vi "Gen - SubPanel Page.vi"(6 "State":T1(ring), 7 "Module Name":string, 8 "Error In":errorcluster, 9 "Module List":string[](array[string]), 10 "Path to Modules Folder":path, 11 "Main SubPanel Ref":refnum<vi>) -> (0 "Error Out":errorcluster)   [LabVIEW 2020]
doc: "Use this VI to calling page and display into subpanel\n\nWriter :\nReader : Main UI"
uses:
  Control/aFGV States - Subpanel.ctl
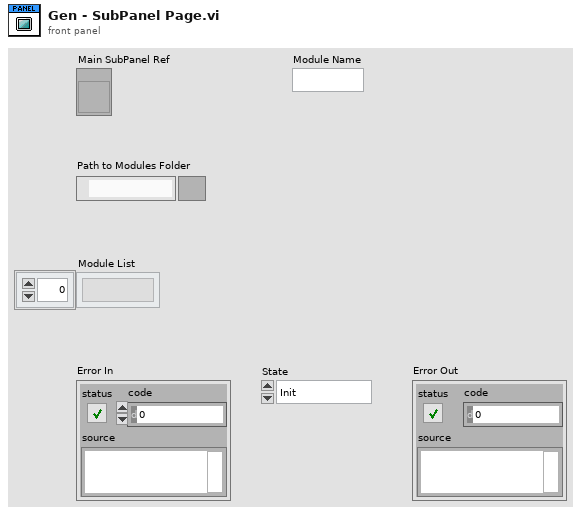
[diagram p1: front panel]
types:
  T1 = enum16{"Init", "Init Module", "Run Module", "Kill Module", "Change Page", "Exit"}
  T2 = typedef "aFGV States - Subpanel.ctl" = enum16{"Init", "Get VI Name", "Update", "Exit"}
  T3 = enum32{"Bad", "Idle", "Run top level", "Running"}
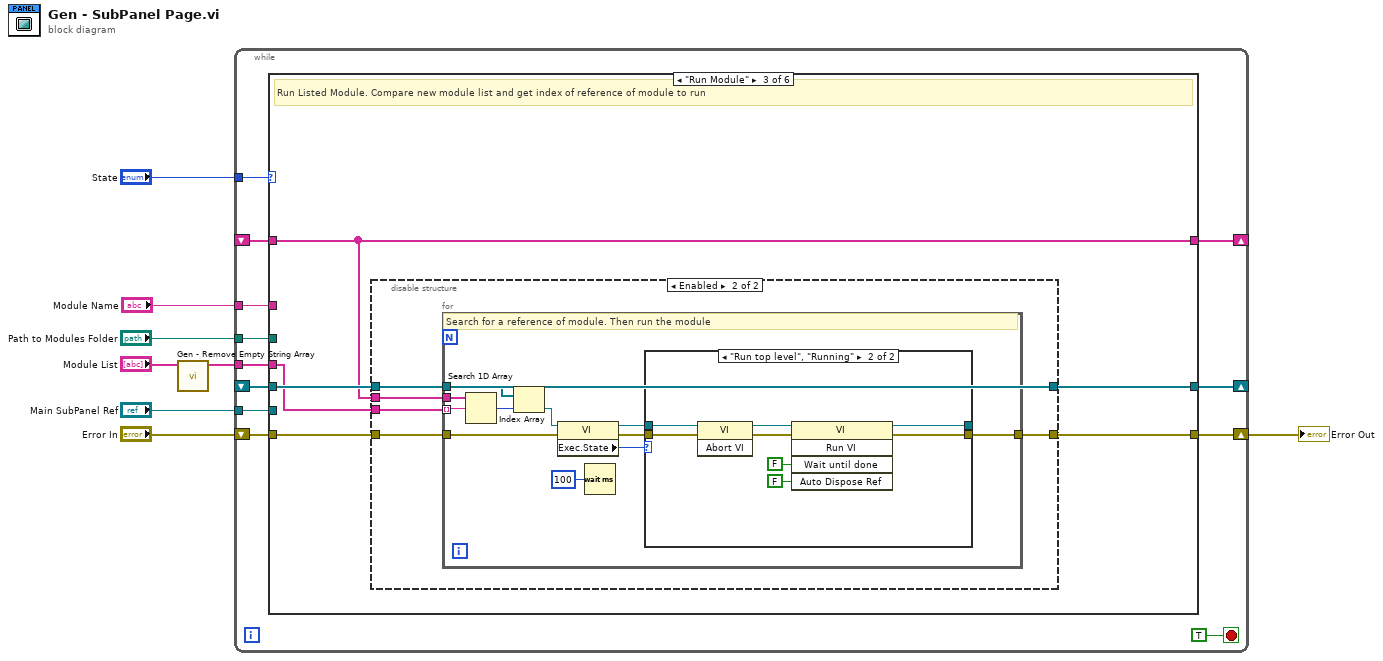
[diagram p0: block diagram]
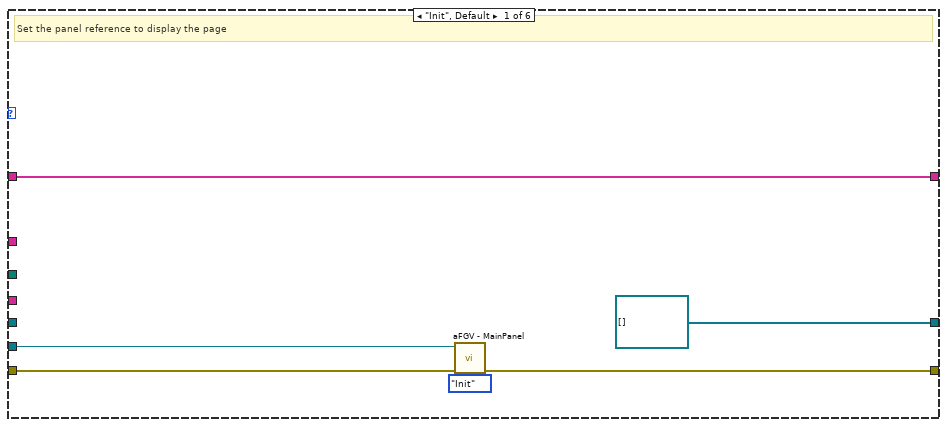
[diagram p2: hidden frame]
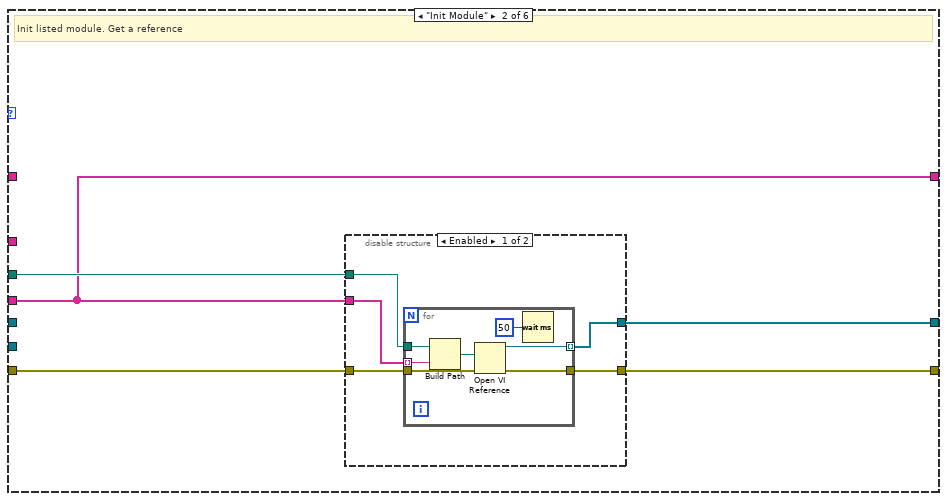
[diagram p3: hidden frame]
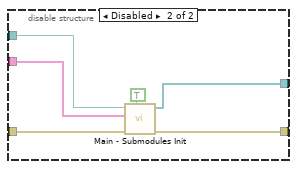
[diagram p4: hidden frame]
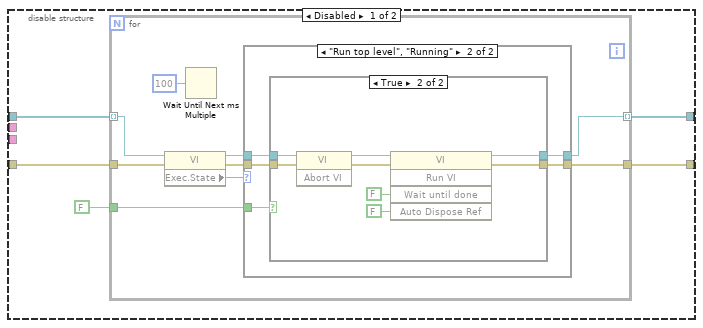
[diagram p5: hidden frame]
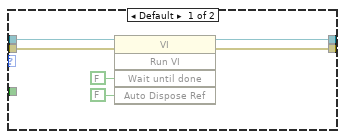
[diagram p6: hidden frame]
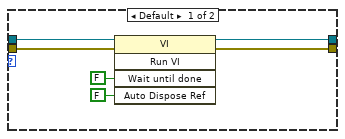
[diagram p8: hidden frame]
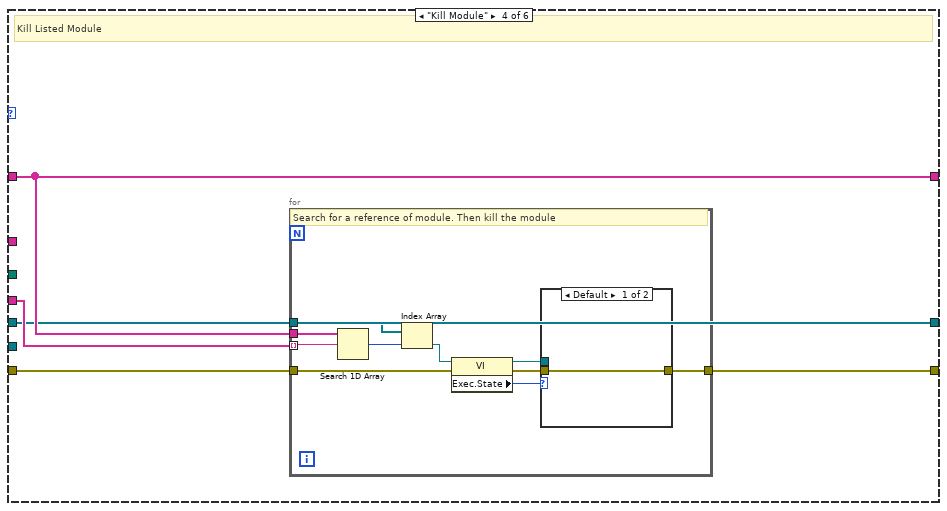
[diagram p9: hidden frame]
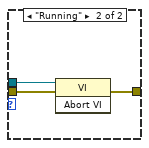
[diagram p10: hidden frame]
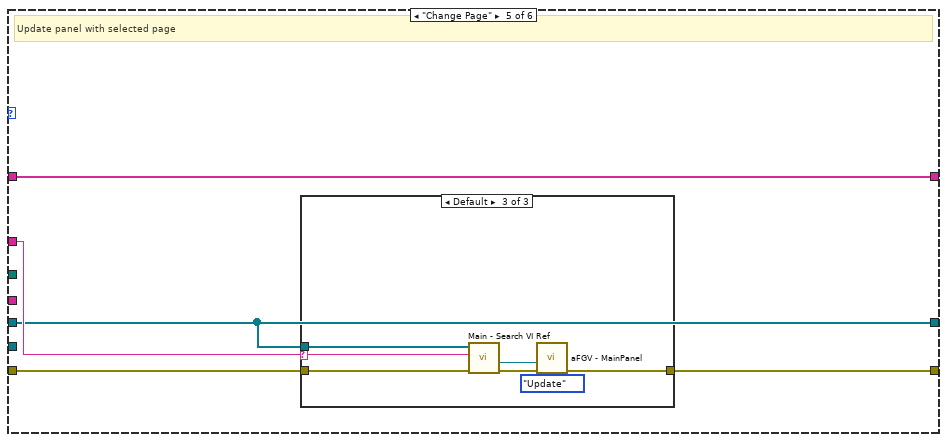
[diagram p11: hidden frame]
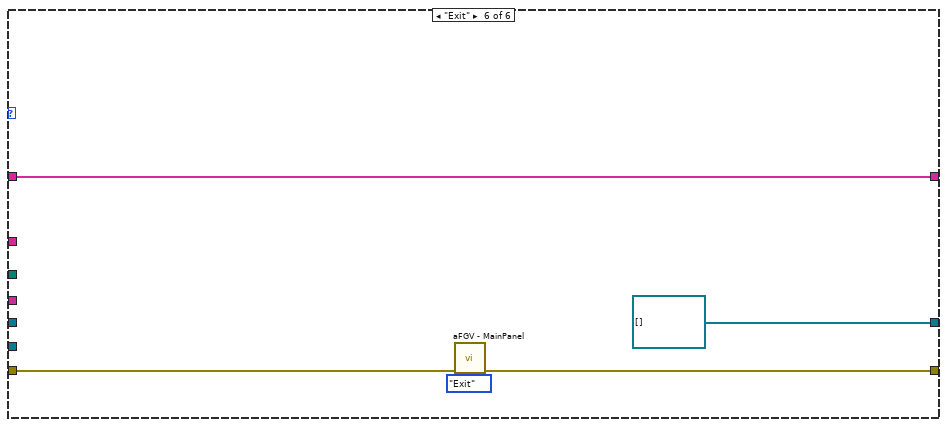
[diagram p14: hidden frame]
diagram:
  n1 = call "Gen - Remove Empty String Array.vi"("Data Array"="Module List") -> ("Data Out"=w2:string[])  [unwired: 10 in]
  n2 = while {
    tunnel: "State" -> [w18]
    tunnel: "Main SubPanel Ref" -> [w17]
    tunnel: "Path to Modules Folder" -> [w16]
    tunnel: w2 -> [w15]
    shift-right: [w19] -> w8
    shift-left: "Error In" -> [w20]
    shift-right: [w13] -> _
    shift-left: _ -> [w11]
    tunnel: "Module Name" -> [w12]
    shift-right: [w10] -> _
    shift-left: _ -> [w9]
    stop <- TRUE stop-if-true
    n3 = case shown="\"Run Module\"" w18 {
      tunnel: [w25 w29 w53 w122 w142 w156] -> w19
      tunnel: w20 -> [w26 w30 w54 w125 w143 w157]
      tunnel: w17 -> [w23 _ _ _ _ _]
      tunnel: w16 -> [_ w31 _ _ _ _]
      tunnel: w15 -> [_ w28 w50 w123 _ _]
      tunnel: [refnum<vi>[] [] ("Module Refnum") w27 w55 w121 w140 refnum<vi>[] [] ("Module Refnum")] -> w13
      tunnel: w12 -> [_ _ _ _ w141 _]
      tunnel: w11 -> [_ _ w52 w121 w140 _]
      tunnel: [w21 w28 w51 w124 w139 w153] -> w10
      tunnel: w9 -> [w21 _ w51 w124 w139 w153]
      frame "Init", Default {
        # "Set the panel reference to display the page"
        n4 = call "aFGV - MainPanel.vi"("Action"=aFGV_States_-_Subpanel."Init", "Error In"=w26, "Main SubPanel Ref"=w23) -> ("Error Out"=w25:errorcluster)  [unwired: 6 in, 2 out]
      }
      frame "Init Module" {
        # "Init listed module. Get a reference"
        n5 = disable-structure shown="Enabled" {
          disable-tunnel: w31 -> [w36 w46]
          disable-tunnel: w28 -> [w35 w47]
          disable-tunnel: w30 -> [w34 w48]
          disable-tunnel: [w33 w45] -> w29
          disable-tunnel: [w32 w44] -> w27
          frame Enabled {
            n6 = for {
              tunnel: w36 -> [w42]
              tunnel: w35 -> [w41] mode=indexing
              tunnel: w34 -> [w40]
              tunnel: [w39] -> w33
              tunnel: [w38] -> w32 mode=indexing
              n7 = Build Path(base path=w42, name or relative path=w41) -> (appended path=w43:path)
              n8 = Open VI Reference(vi path=w43, error in (no error)=w40) -> (vi reference=w38:refnum<vi>, error out=w39:errorcluster)  [unwired: 4 in]
              n9 = Wait (ms)(milliseconds to wait=u32 50) -> ()  [unwired: 1 out]
            }
          }
          frame Disabled {
            n10 = call "Main - Submodules Init.vi"("Kill if running?"=TRUE, "Error In"=w48, "VIs name"=w47, "Path to Modules Folder"=w46) -> ("Error Out"=w45:errorcluster, "Module Refnum"=w44:refnum<vi>[])  [unwired: 6 in]
          }
        }
      }
      frame "Run Module" {
        # "Run Listed Module. Compare new module list and get index of reference of module to run"
        n11 = disable-structure shown="Enabled" {
          disable-tunnel: [w60 w95] -> w55
          disable-tunnel: w54 -> [w59 w92]
          disable-tunnel: [w58 w91] -> w53
          disable-tunnel: w52 -> [w56 w95]
          disable-tunnel: w51 -> [_ w94]
          disable-tunnel: w50 -> [_ w93]
          frame Disabled {
            n12 = for {
              tunnel: w59 -> [w69]
              tunnel: [w67] -> w58
              tunnel: [w62] -> w60 mode=indexing
              tunnel: FALSE ("Kill if running?") -> [w64]
              tunnel: w56 -> [w61] mode=indexing
              n13 = property class="VI"(reference=w61, error in=w69) -> (reference out=w65:refnum<vi>, error out=w68:errorcluster, "Exec.State"=w66:T3)
              n14 = Wait Until Next ms Multiple(millisecond multiple=u32 100) -> ()  [unwired: 1 out]
              n15 = case shown="\"Run top level\", \"Running\"" w66 {
                tunnel: w68 -> [w75 w80]
                tunnel: w65 -> [w71 w78]
                tunnel: [w70 w77] -> w62
                tunnel: [w74 w79] -> w67
                tunnel: w64 -> [_ w76]
                frame Default {
                  n16 = invoke class="VI" method="Run VI"(reference=w71, error in=w75, "Wait until done"=FALSE ("Wait Until Done"), "Auto Dispose Ref"=FALSE ("Auto Dispose Reference")) -> (reference out=w70:refnum<vi>, error out=w74:errorcluster)  [unwired: 1 in, 3 out]
                }
                frame "Run top level", "Running" {
                  n17 = case shown="True" w76 {
                    tunnel: w80 -> [w82 w90]
                    tunnel: w78 -> [w81 w87]
                    tunnel: [w81 w83] -> w77
                    tunnel: [w82 w88] -> w79
                    frame False {
                    }
                    frame True {
                      n18 = invoke class="VI" method="Abort VI"(reference=w87, error in=w90) -> (reference out=w84:refnum<vi>, error out=w89:errorcluster)  [unwired: 1 in, 1 out]
                      n19 = invoke class="VI" method="Run VI"(reference=w84, error in=w89, "Wait until done"=FALSE ("Wait Until Done"), "Auto Dispose Ref"=FALSE ("Auto Dispose Reference")) -> (reference out=w83:refnum<vi>, error out=w88:errorcluster)  [unwired: 1 in, 3 out]
                    }
                  }
                }
              }
            }
          }
          frame Enabled {
            n20 = for {
              tunnel: w94 -> [w106]
              tunnel: w93 -> [w105] mode=indexing
              tunnel: [w99] -> w91
              tunnel: w92 -> [w102]
              tunnel: w95 -> [w104]
              # "Search for a reference of module. Then run the module"
              n21 = Search 1D Array(1D array=w106, element=w105) -> (index of element=w103:i32)  [unwired: 1 in]
              n22 = Index Array(array=w104, index=w103) -> (element=w101:refnum<vi>)
              n23 = property class="VI"(reference=w101, error in=w102) -> (reference out=w98:refnum<vi>, error out=w100:errorcluster, "Exec.State"=w97:T3)
              n24 = Wait (ms)(milliseconds to wait=u32 100) -> ()  [unwired: 1 out]
              n25 = case shown="\"Run top level\", \"Running\"" w97 {
                tunnel: w100 -> [w112 w120]
                tunnel: w98 -> [w108 w118]
                tunnel: [w107 w117] -> _
                tunnel: [w111 w119] -> w99
                frame Default {
                  n26 = invoke class="VI" method="Run VI"(reference=w108, error in=w112, "Wait until done"=FALSE ("Wait Until Done"), "Auto Dispose Ref"=FALSE ("Auto Dispose Reference")) -> (reference out=w107:refnum<vi>, error out=w111:errorcluster)  [unwired: 1 in, 3 out]
                }
                frame "Run top level", "Running" {
                  n27 = invoke class="VI" method="Abort VI"(reference=w118, error in=w120) -> (reference out=w113:refnum<vi>, error out=w116:errorcluster)  [unwired: 1 in, 1 out]
                  n28 = invoke class="VI" method="Run VI"(reference=w113, error in=w116, "Wait until done"=FALSE ("Wait Until Done"), "Auto Dispose Ref"=FALSE ("Auto Dispose Reference")) -> (reference out=w117:refnum<vi>, error out=w119:errorcluster)  [unwired: 1 in, 3 out]
                }
              }
            }
          }
        }
      }
      frame "Kill Module" {
        # "Kill Listed Module"
        n29 = for {
          tunnel: w124 -> [w134]
          tunnel: w123 -> [w133] mode=indexing
          tunnel: [w131] -> w122
          tunnel: w125 -> [w129]
          tunnel: w121 -> [w132]
          # "Search for a reference of module. Then kill the module"
          n30 = Search 1D Array(1D array=w134, element=w133) -> (index of element=w130:i32)  [unwired: 1 in]
          n31 = Index Array(array=w132, index=w130) -> (element=w128:refnum<vi>)
          n32 = property class="VI"(reference=w128, error in=w129) -> (error out=w127:errorcluster, "Exec.State"=w126:T3)  [unwired: 1 out]
          n33 = case shown="Default" w126 {
            tunnel: [w135 w138] -> w131
            tunnel: w128 -> [_ w137]
            tunnel: w127 -> [w135 w136]
            frame Default {
            }
            frame "Running" {
              n34 = invoke class="VI" method="Abort VI"(reference=w137, error in=w136) -> (error out=w138:errorcluster)  [unwired: 1 in, 2 out]
            }
          }
        }
      }
      frame "Change Page" {
        # "Update panel with selected page"
        n35 = case shown="Default" w141 {
          selector: w141 -> [_ _ w146]
          tunnel: w143 -> [w144 w145 w148]
          tunnel: [w144 w145 w151] -> w142
          tunnel: w140 -> [_ _ w147]
          frame "<>" {
          }
          frame "0" {
          }
          frame Default {
            n36 = call "Main - Search VI Ref.vi"("Error In"=w148, "VI Name to Search"=w146, "VI Refs"=w147) -> ("Error Out"=w152:errorcluster, "VI Ref Found"=w150:refnum<vi>)  [unwired: 7 in]
            n37 = call "aFGV - MainPanel.vi"("Action"=aFGV_States_-_Subpanel."Update", "Error In"=w152, "VI Ref"=w150) -> ("Error Out"=w151:errorcluster)  [unwired: 6 in, 2 out]
          }
        }
      }
      frame "Exit" {
        n38 = call "aFGV - MainPanel.vi"("Action"=aFGV_States_-_Subpanel."Exit", "Error In"=w157) -> ("Error Out"=w156:errorcluster)  [unwired: 7 in, 2 out]
      }
    }
  }
  "Error Out" <- w8
